vi "ASI_serial_test.vi"() -> ()   [LabVIEW 2012]
uses:
  <vilib>/Instr/_visa.llb/VISA Configure Serial Port (Instr).vi
panel:
  in  "Character to append":string
  in  "milliseconds to wait":u32=5
  in  "Send Hex":bool
  out "Command Hex":string
  out "ASCII output":string
  out "value":i16
  in  "Hex input string":string
  in  "Convert Hex to ASCII":bool
  out "Current Z position (um)":dbl
  in  "Read Z":bool
  in  "Z position (um)":dbl
  in  "Move to":bool
  out "Serial Settings:Number of Bytes at Serial Port TIME OUT":u32
  in  "Read":bool
  out "return count":u32
  out "error out":errorcluster
  out "Number of Bytes at Serial Port":u32
  out "Read buffer":string
  in  "Command":string
  in  "Send":bool
  in  "stop":bool
  out "VISA resource name out":refnum<visa-resource-name>
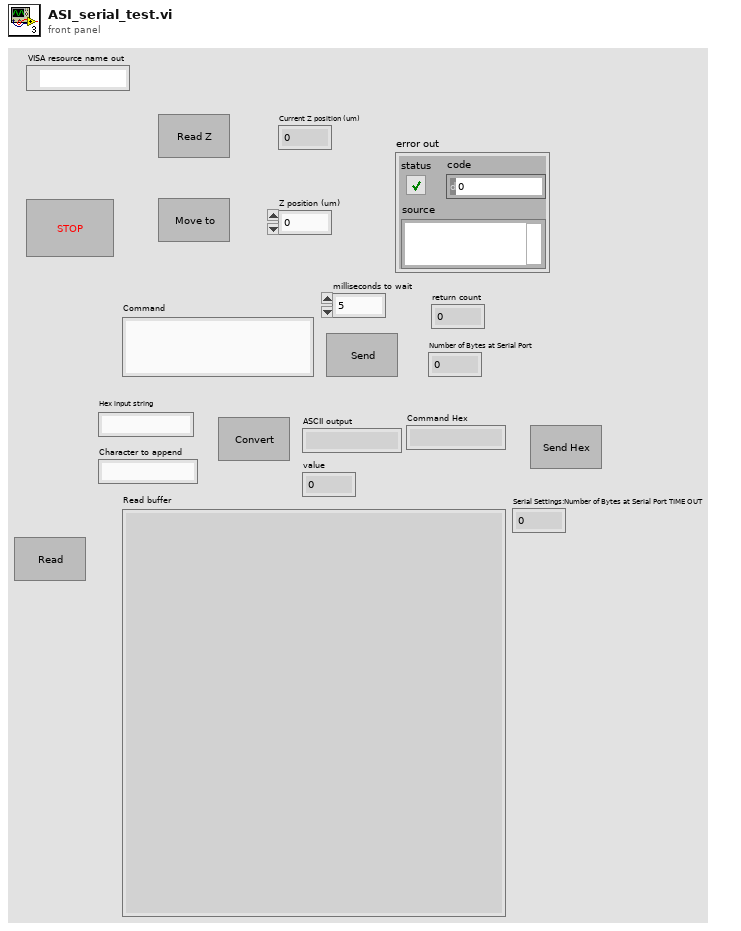
[diagram p1: front panel]
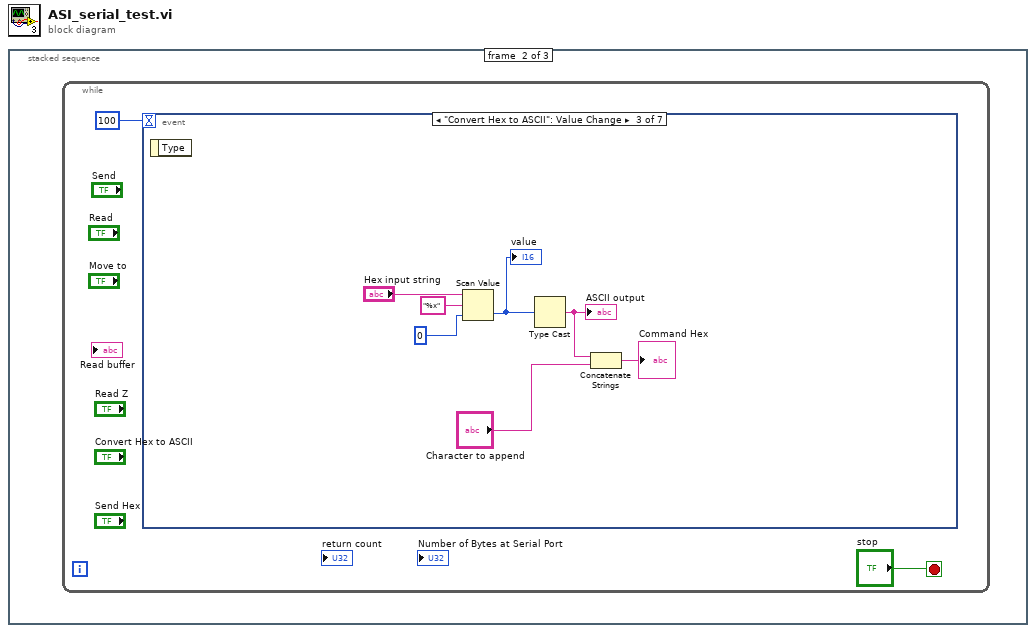
[diagram p0: block diagram]
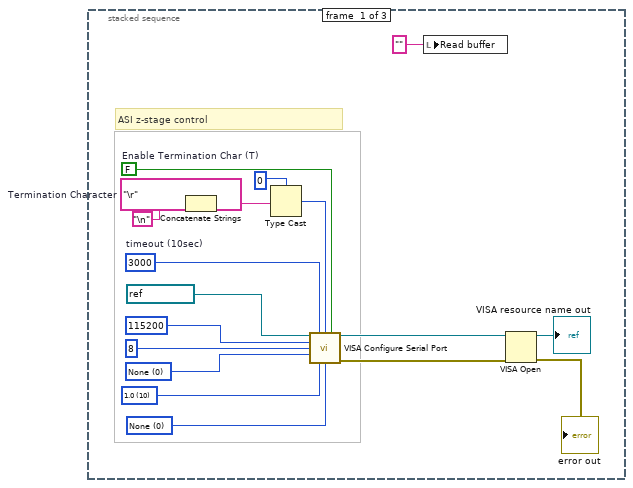
[diagram p2: hidden frame]
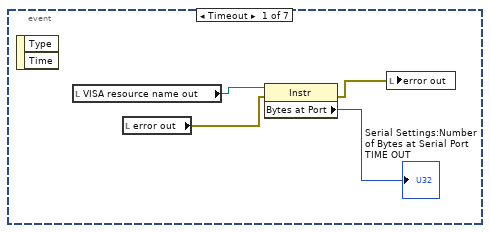
[diagram p3: hidden frame]
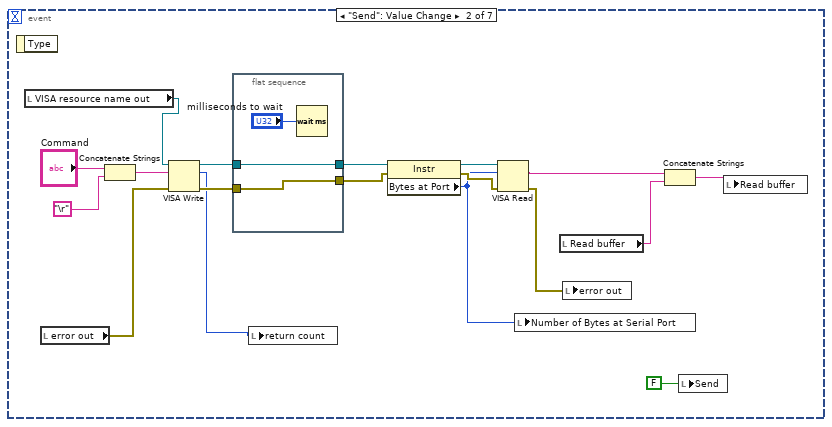
[diagram p4: hidden frame]
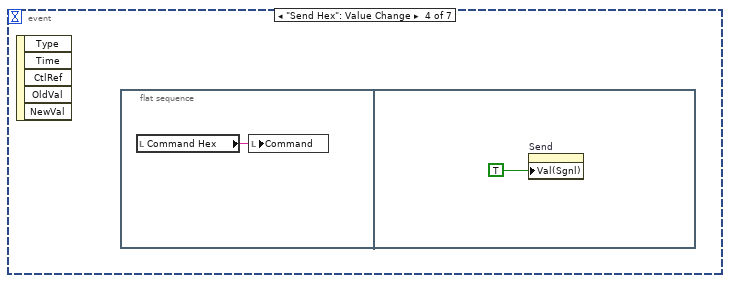
[diagram p5: hidden frame]
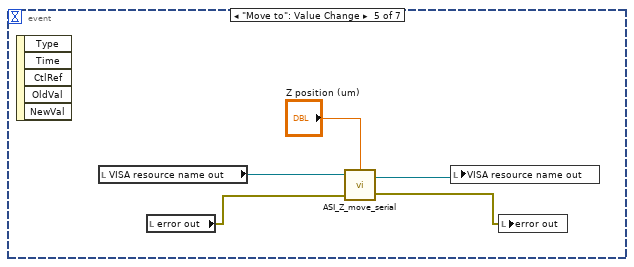
[diagram p6: hidden frame]
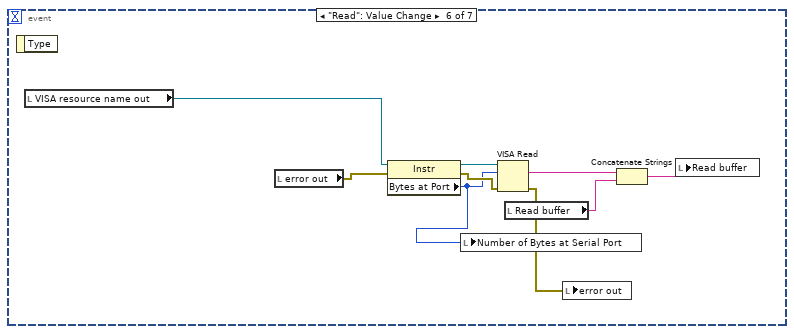
[diagram p7: hidden frame]
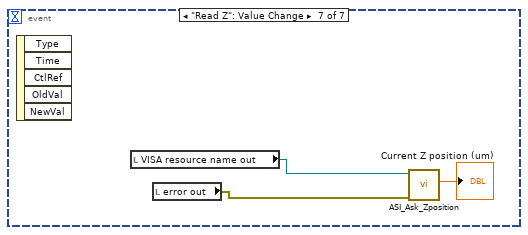
[diagram p8: hidden frame]
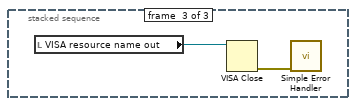
[diagram p9: hidden frame]
diagram:
  n1 = stacked-sequence {
    frame #0 {
      w5 = u16 0 items=["None"=0, "XON/XOFF"=1, "RTS/CTS"=2, "DTR/DSR"=4] ("flow control")
      w15 = u16 10 items=["1.0"=10, "1.5"=15, "2.0"=20] ("stop bits")
      w12 = u16 0 items=["None", "Odd", "Even", "Mark", "Space"] ("parity")
      w9 = "\r"  # Termination Character
      w14 = FALSE  # Enable Termination Char (T)
      w13 = u32 3000  # timeout (10sec)
      # "ASI z-stage control"
      n2 = Concatenate Strings(w9, "\n") -> (w7:string)
      n3 = Type Cast(type=u8 0, x=w7) -> (*(type *) &x=w18:u8)
      n4 = call-poly "VISA Configure Serial Port"("VISA resource name"=refnum<visa-resource-name> "COM17" ("COM17"), "timeout (10sec)"=w13, "termination char\n(0xA = '\\n' = LF)"=w18, "Enable Termination\nChar (T)"=w14, "baud rate (9600)"=u32 115200 ("baud rate"), "data bits (8)"=u16 8 ("data bits"), "parity (0:none)"=w12, "stop bits (10: 1 bit)"=w15, "flow control (0:none)"=w5) -> ("VISA resource name out"=w6:refnum<visa-resource-name>, "error out"=w3:errorcluster)  [unwired: 5 in]
      n5 = local write "Read buffer"("" ("Read buffer")) -> ()
      n6 = VISA Open(error in (no error)=w3, VISA resource name=w6) -> (VISA resource name=→"VISA resource name out":refnum<visa-resource-name>, error out=→"error out":errorcluster)  [unwired: 3 in]
    }
    frame #1 {
      n7 = while {
        stop <- "stop" stop-if-true
        n8 = event shown="[2] \"Convert Hex to ASCII\": Value Change" {
          selector: _ -> [_ _ _ _ _ _ _]
          dyn-events: _ -> [_ _ _ _ _ _ _]
          timeout: 100 -> [_ _ _ _ _ _ _]
          event Timeout {
            n9 = event-data() -> ()  [unwired: 1 in, 2 out]
            n10 = local read "VISA resource name out"() -> (w24:refnum<visa-resource-name>)
            n11 = local read "error out"() -> (w22:errorcluster)
            n12 = property class="Instr"(reference=w24, error in=w22) -> (error out=w21:errorcluster, "Bytes at Port"=→"Serial Settings:Number of Bytes at Serial Port TIME OUT":u32)  [unwired: 1 out]
            n13 = local write "error out"(w21) -> ()
          }
          event "Send": Value Change {
            n14 = event-data() -> ()  [unwired: 1 in, 1 out]
            n15 = local read "VISA resource name out"() -> (w42:refnum<visa-resource-name>)
            n16 = local read "error out"() -> (w38:errorcluster)
            n17 = Concatenate Strings("Command", "\r") -> (w31:string)
            n18 = VISA Write(VISA resource name=w42, write buffer=w31, error in (no error)=w38) -> (VISA resource name out=w41:refnum<visa-resource-name>, return count=w28:u32, error out=w36:errorcluster)
            n19 = flat-sequence {
              tunnel: [w45] -> w40
              tunnel: w41 -> [w45]
              tunnel: [w44] -> w37
              tunnel: w36 -> [w44]
              frame #0 {
                n20 = Wait (ms)(milliseconds to wait="milliseconds to wait") -> ()  [unwired: 1 out]
              }
            }
            n21 = local write "return count"(w28) -> ()
            n22 = property class="Instr"(reference=w40, error in=w37) -> (reference out=w39:refnum<visa-resource-name>, error out=w35:errorcluster, "Bytes at Port"=w27:u32)
            n23 = VISA Read(VISA resource name=w39, byte count=w27, error in (no error)=w35) -> (read buffer=w29:string, error out=w34:errorcluster)  [unwired: 2 out]
            n24 = local write "Number of Bytes at Serial Port"(w27) -> ()
            n25 = local read "Read buffer"() -> (w26:string)
            n26 = local write "error out"(w34) -> ()
            n27 = Concatenate Strings(w29, w26) -> (w30:string)
            n28 = local write "Send"(FALSE ("Send")) -> ()
            n29 = local write "Read buffer"(w30) -> ()
          }
          event "Convert Hex to ASCII": Value Change {
            n30 = event-data() -> ()  [unwired: 1 in, 1 out]
            n31 = Scan Value(string="Hex input string", format string="%x", default (0 dbl)=i16 0) -> (value=w49:i16)  [unwired: 1 out]
            "value" <- w49
            n32 = Type Cast(x=w49) -> (*(type *) &x=w48:string)  [unwired: 1 in]
            "ASCII output" <- w48
            n33 = Concatenate Strings(w48, "Character to append") -> (→"Command Hex":string)
          }
          event "Send Hex": Value Change {
            n34 = event-data() -> ()  [unwired: 1 in, 5 out]
            n35 = flat-sequence {
              frame #0 {
                n36 = local read "Command Hex"() -> (w53:string)
                n37 = local write "Command"(w53) -> ()
              }
              frame #1 {
                n38 = property on="Send" class="Bool (strict)"("Val(Sgnl)"=TRUE ("Send")) -> ()  [unwired: 2 in, 2 out]
              }
            }
          }
          event "Move to": Value Change {
            n39 = event-data() -> ()  [unwired: 1 in, 5 out]
            n40 = local read "VISA resource name out"() -> (w59:refnum<visa-resource-name>)
            n41 = local read "error out"() -> (w58:errorcluster)
            n42 = call "ASI_Z_move_serial.vi"("Z position (um)"="Z position (um)", "error in"=w58, "VISA resource name"=w59) -> ("error out"=w55:errorcluster, "VISA resource name out"=w56:refnum<visa-resource-name>)  [unwired: 1 in]
            n43 = local write "VISA resource name out"(w56) -> ()
            n44 = local write "error out"(w55) -> ()
          }
          event "Read": Value Change {
            n45 = event-data() -> ()  [unwired: 1 in, 1 out]
            n46 = local read "VISA resource name out"() -> (w65:refnum<visa-resource-name>)
            n47 = local read "error out"() -> (w64:errorcluster)
            n48 = property class="Instr"(reference=w65, error in=w64) -> (reference out=w68:refnum<visa-resource-name>, error out=w67:errorcluster, "Bytes at Port"=w63:u32)
            n49 = local write "Number of Bytes at Serial Port"(w63) -> ()
            n50 = VISA Read(VISA resource name=w68, byte count=w63, error in (no error)=w67) -> (read buffer=w61:string, error out=w66:errorcluster)  [unwired: 2 out]
            n51 = local read "Read buffer"() -> (w60:string)
            n52 = local write "error out"(w66) -> ()
            n53 = Concatenate Strings(w61, w60) -> (w62:string)
            n54 = local write "Read buffer"(w62) -> ()
          }
          event "Read Z": Value Change {
            n55 = event-data() -> ()  [unwired: 1 in, 5 out]
            n56 = local read "VISA resource name out"() -> (w71:refnum<visa-resource-name>)
            n57 = local read "error out"() -> (w70:errorcluster)
            n58 = call "ASI_Ask_Zposition.vi"("error in"=w70, "VISA resource name"=w71) -> ("Current Z position (um)"=→"Current Z position (um)":dbl)  [unwired: 7 in, 2 out]
          }
        }
      }
    }
    frame #2 {
      n59 = local read "VISA resource name out"() -> (w72:refnum<visa-resource-name>)
      n60 = VISA Close(VISA resource name=w72) -> (error out=w73:errorcluster)  [unwired: 1 in]
      n61 = call <vilib>:"Simple Error Handler.vi"("error in (no error)"=w73) -> ()  [unwired: 4 in, 5 out]
    }
  }
